vi "search hierarchy.vi"(10 "ID":string, 11 "hierarchy":T1[](array[typedef])) -> (3 "index":i32)   [LabVIEW 2025, in "CEF.lvlib"]
doc: "Searches a hierarchy set for a given ID and returns its index.Copyright 2017 National Instruments Corporation\n\nLicensed under the Apache License, Version 2.0 (the \"License\"); you may not use this file except in compliance with the License. You may obtain a copy of the License at http://www.apache.org/licenses/LICENSE-2.0\nUnless required by applicable law or agreed to in writing, software distributed under the License is distributed on an \"AS IS\" BASIS, WITHOUT WARRANTIES OR CONDITIONS OF ANY KIND, either express or implied. See the License for the specific language governing permissions and limitations under the License."
uses:
  CEF.lvlib
  hierarchy element.ctl
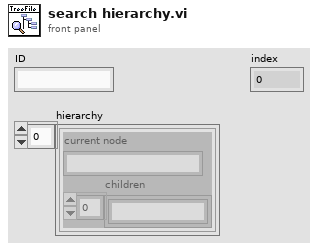
[diagram p1: front panel]
types:
  T1 = typedef "CEF.lvlib/hierarchy element.ctl" = cluster{"current node":string, "children":string[]}
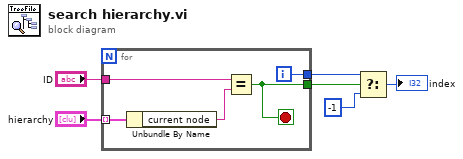
[diagram p0: block diagram]
diagram:
  n1 = for {
    tunnel: "hierarchy" -> [w11] mode=indexing
    tunnel: "ID" -> [w9]
    tunnel: [w7] -> w4
    tunnel: [w8] -> w3
    i -> [w8]
    stop <- w7 stop-if-true
    n2 = Unbundle By Name(w11) -> ("current node"=w10:string)
    n3 = Equal?(x=w9, y=w10) -> (x = y?=w7:bool)
  }
  n4 = Select(t=w3, s=w4, f=-1) -> (s? t:f=→"index":i32)
